vi "ReadModeNew.vi"() -> ()   [LabVIEW 2022 SP3]
uses:
  Haptic-Programming-Interface/LabVIEW VIs/Haptic Prog Interface/Haptic Prog Interface.lvlib
  <userlib>/Nanonis Prog Interface V5/Nanonis Prog Interface.lvlib
panel:
  out "Z position (m)":sgl format="%#_6p"
  out "Center coordinates (m)":cluster{"Xc":sgl, "Yc":sgl} {"Yc" format="%.2p"; "Xc" format="%.2p"}
  out "Size (m)":cluster{"Width":sgl, "Height":sgl} {"Height" format="%.2p"; "Width" format="%.2p"}
  out "Angle (deg)":sgl format="%.2f"
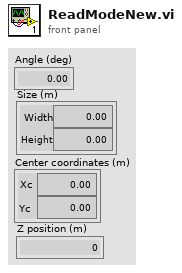
[diagram p1: front panel]
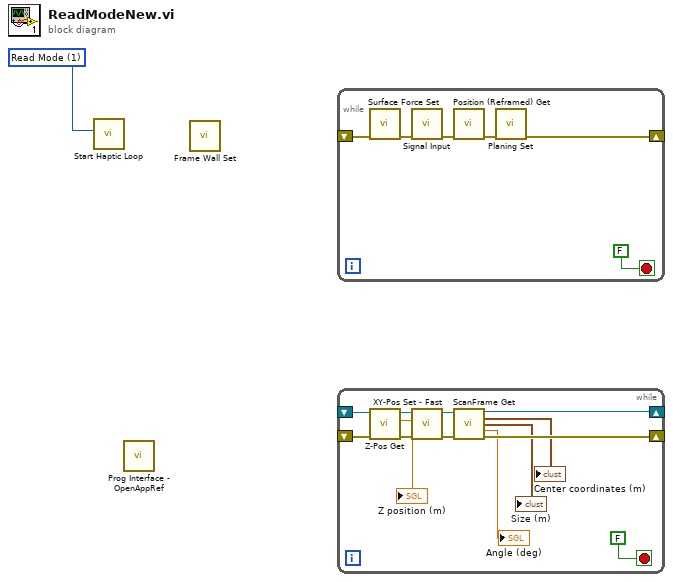
[diagram p0: block diagram]
diagram:
  w1 = u16 1 items=["Custom Mode", "Read Mode", "Write Mode"] ("Mode Selection")
  n1 = call <userlib>:"Start Haptic Loop.vi"("Mode Selection"=w1) -> ()  [unwired: 10 in, 1 out]
  n2 = call <userlib>:"Prog Interface - OpenAppRef.vi"() -> ()  [unwired: 6 in, 2 out]
  n3 = call <userlib>:"Frame Wall Set.vi"() -> ()  [unwired: 11 in, 1 out]
  n4 = while {
    shift-right: [w2] -> _
    shift-left: _ -> [w3]
    stop <- FALSE stop-if-true
    n5 = call <userlib>:"Surface Force Set.vi"("error in (no error)"=w3) -> ("error out"=w6:errorcluster)  [unwired: 10 in]
    n6 = call <userlib>:"Signal Input.vi"("error in (no error)"=w6) -> ("error out"=w5:errorcluster)  [unwired: 10 in]
    n7 = call <userlib>:"Position (Reframed) Get.vi"("error in (no error)"=w5) -> ("error out"=w4:errorcluster)  [unwired: 13 in, 1 out]
    n8 = call <userlib>:"Planing Set.vi"("error in (no error)"=w4) -> ("error out"=w2:errorcluster)  [unwired: 9 in, 1 out]
  }
  n9 = while {
    shift-right: [w16] -> _
    shift-left: _ -> [w19]
    shift-right: [w9] -> _
    shift-left: _ -> [w12]
    stop <- FALSE stop-if-true
    n10 = call <userlib>:"Z-Pos Get.vi"("error in (no error)"=w19, "Application ref in"=w12) -> ("error out"=w18:errorcluster, "Z position (m)"=→"Z position (m)":sgl, "Application ref out"=w11:refnum<vi>)  [unwired: 7 in]
    n11 = call <userlib>:"XY-Pos Set - Fast.vi"("error in (no error)"=w18, "Application ref in"=w11) -> ("error out"=w17:errorcluster, "Application ref out"=w10:refnum<vi>)  [unwired: 7 in]
    n12 = call <userlib>:"ScanFrame Get.vi"("Application ref in"=w10, "error in (no error)"=w17) -> ("Application ref out"=w9:refnum<vi>, "Center coordinates (m)"=→"Center coordinates (m)":cluster{"Xc":sgl, "Yc":sgl}, "Size (m)"=→"Size (m)":cluster{"Width":sgl, "Height":sgl}, "Angle (deg)"=→"Angle (deg)":sgl, "error out"=w16:errorcluster)  [unwired: 9 in]
  }
